vi "Tree.Initialize.vi"(8 "error in (no error)":errorcluster, 10 "Tree Strings":string[](array[string]), 11 "TreeControl":refnum<vi>) -> (0 "error out":errorcluster, 3 "TreeControl out":refnum<vi>)   [LabVIEW 2014, in "NIAnalysis.lvlib"]
uses:
  NIAnalysis.lvlib
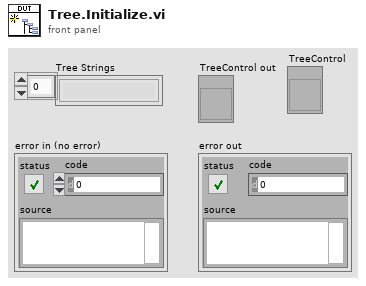
[diagram p1: front panel]
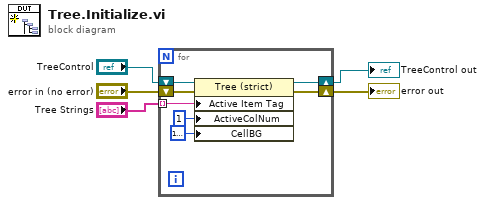
[diagram p0: block diagram]
diagram:
  n1 = for {
    tunnel: "Tree Strings" -> [w9] mode=indexing
    shift-right: [w8] -> w5
    shift-left: "TreeControl" -> [w10]
    shift-right: [w6] -> w4
    shift-left: "error in (no error)" -> [w7]
    n2 = property class="Tree (strict)"(reference=w10, error in=w7, "Active Item Tag"=w9, "ActiveColNum"=1 ("Active Cell:Active Column Number"), "CellBG"=u32 16777216) -> (reference out=w8:refnum<vi>, error out=w6:errorcluster)
  }
  "TreeControl out" <- w5
  "error out" <- w4
